vi "Parallel Event Init.vi"(5 "stop":refnum<vi>, 6 "parent":refnum<vi>, 7 "error in":errorcluster, 8 "max PVs per thread":i32=100, 9 "field names":string[](array[string]), 10 "PV names":string[](array[string])) -> (0 "error out":errorcluster, 1 "number of threads":i32, 2 "references of results":T1(array[cluster]), 3 "subVI References":cluster{refnum<vi>[], refnum<vi>[]})   [LabVIEW 2019]
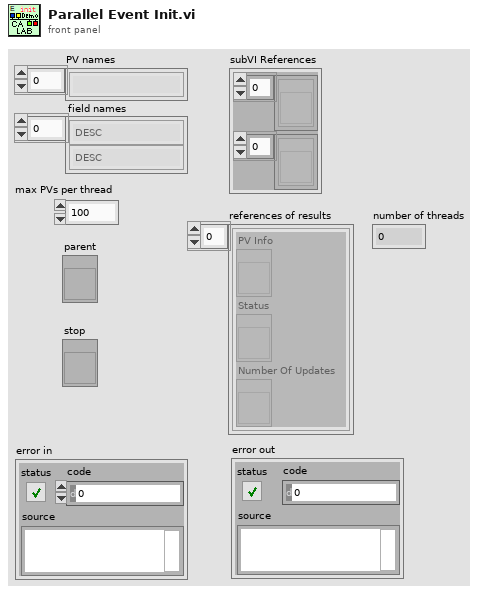
[diagram p1: front panel]
types:
  T1 = cluster{"PV Info":refnum<vi>, "Status":refnum<vi>, "Number Of Updates":refnum<vi>}[]
  T2 = map{string, cluster{"PV Info":refnum<vi>, "Status":refnum<vi>, "Number Of Updates":refnum<vi>}}
  T3 = cluster{"PV Info":refnum<vi>, "Status":refnum<vi>, "Number Of Updates":refnum<vi>}
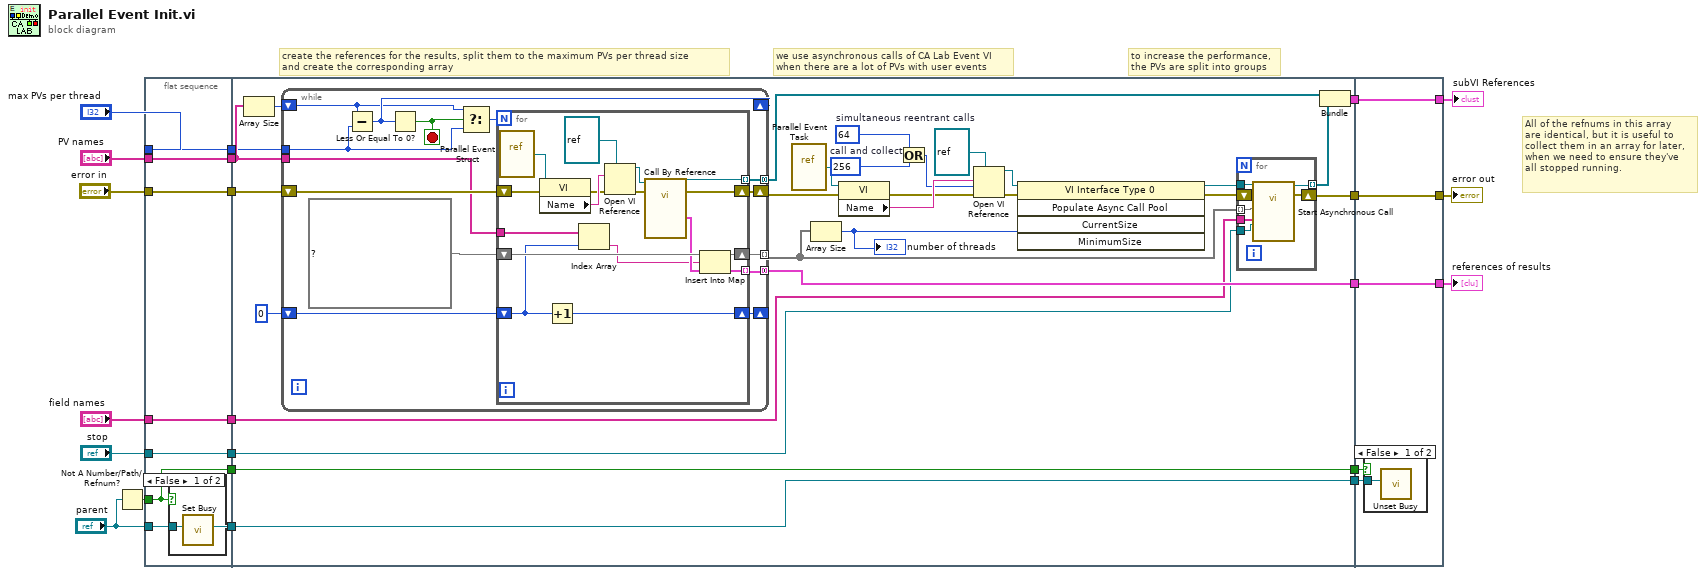
[diagram p0: block diagram]
diagram:
  # "All of the refnums in this array\nare identical, but it is useful to\ncollect them in an array for later,\nwhen we need to ensure they've\nall stopped running."
  # "create the references for the results, split them to the maximum PVs per thread size\nand create the corresponding array"
  # "to increase the performance,\nthe PVs are split into groups"
  # "we use asynchronous calls of CA Lab Event VI\nwhen there are a lot of PVs with user events"
  n1 = Not A Number/Path/Refnum?(number/path/refnum="parent") -> (NaN/Path/Refnum?=w3:bool)
  n2 = flat-sequence {
    tunnel: "field names" -> [w25]
    tunnel: "stop" -> [w26]
    tunnel: "max PVs per thread" -> [w27]
    tunnel: "PV names" -> [w28]
    tunnel: "error in" -> [w29]
    tunnel: [w29] -> w14
    tunnel: [w28] -> w13
    tunnel: [w27] -> w12
    tunnel: [w26] -> w11
    tunnel: [w25] -> w10
    tunnel: "parent" -> [w24]
    tunnel: [w24] -> w5
    tunnel: w3 -> [w23]
    tunnel: [w23] -> w1
    tunnel: w14 -> [w58]
    tunnel: w13 -> [w40]
    tunnel: w12 -> [w38]
    tunnel: w11 -> [w37]
    tunnel: w10 -> [w35]
    tunnel: [w43] -> w9
    tunnel: [w42] -> w8
    tunnel: [w33] -> w7
    tunnel: [w32] -> w6
    tunnel: w5 -> [w32]
    tunnel: [w31] -> w2
    tunnel: w1 -> [w31]
    tunnel: [w98] -> w15
    tunnel: [w99] -> w20
    tunnel: [w100] -> w21
    tunnel: w9 -> [w100]
    tunnel: w8 -> [w99]
    tunnel: w7 -> [w98]
    tunnel: w6 -> [w97]
    tunnel: w2 -> [w96]
    frame #0 {
      n3 = case shown="False" w23 {
        tunnel: w24 -> [w30 _]
        frame False {
          n4 = call <vilib>:"Set Busy.vi"("VI reference (current VI)"=w30) -> ()  [unwired: 9 in, 2 out]
        }
        frame True {
        }
      }
    }
    frame #1 {
      w48 = 256  # call and collect
      w49 = 64  # simultaneous reentrant calls
      n5 = Array Size(array=w40) -> (size(s)=w39:i32)
      n6 = while {
        tunnel: [w78] -> w36 mode=concatenating
        shift-right: [w77] -> w34
        shift-left: w58 -> [w79]
        tunnel: [w76] -> w44 mode=indexing
        shift-right: [w74] -> _
        shift-left: 0 -> [w75]
        shift-right: [w70] -> _
        shift-left: w39 -> [w68]
        tunnel: [w72] -> w43 mode=concatenating
        tunnel: w40 -> [w67]
        tunnel: w38 -> [w66]
        stop <- w69 stop-if-true
        n7 = Subtract(x=w68, y=w66) -> (x-y=w70:i32)
        n8 = Less Or Equal To 0?(x=w70) -> (x <= 0?=w69:bool)
        n9 = Select(t=w68, s=w69, f=w66) -> (s? t:f=w71:i32)
        n10 = for {
          N: w71 -> [_]
          tunnel: [w89] -> w78 mode=indexing
          shift-right: [w88] -> w77
          shift-left: w79 -> [w87]
          shift-right: [w86] -> w76
          shift-left: T2 {} ("map in") -> [w85]
          shift-right: [w80] -> w74
          shift-left: w75 -> [w83]
          tunnel: [w84] -> w72 mode=indexing
          tunnel: w67 -> [w81]
          n11 = vi-ref "Parallel Event Struct.vi"() -> (w95:refnum<vi>)
          n12 = property class="VI"(reference=w95, error in=w87) -> (error out=w90:errorcluster, "Name"=w94:string)  [unwired: 1 out]
          n13 = Increment(x=w83) -> (x+1=w80:i32)
          n14 = Index Array(array=w81, index=w83) -> (element=w82:string)
          n15 = Open VI Reference(type specifier VI Refnum (for type only)=refnum<vi> refnum, vi path=w94, error in (no error)=w90) -> (vi reference=w92:refnum<vi>, error out=w91:errorcluster)  [unwired: 3 in]
          n16 = call-by-ref "?"(reference=w92, error in=w91) -> (reference out=w89:refnum<vi>, error out=w88:errorcluster, "References"=w84:T3)
          n17 = Insert Into Map(map in=w85, key=w82, value=w84) -> (map out=w86:T2)  [unwired: 2 out]
        }
      }
      n18 = vi-ref "Parallel Event Task.vi"() -> (w56:refnum<vi>)
      n19 = Array Size(array=w44) -> (size(s)=w50:i32)
      "number of threads" <- w50
      n20 = property class="VI"(reference=w56, error in=w34) -> (error out=w54:errorcluster, "Name"=w55:string)  [unwired: 1 out]
      n21 = Or(x=w49, y=w48) -> (x .or. y?=w47:i32)
      n22 = Open VI Reference(type specifier VI Refnum (for type only)=refnum<vi> refnum, vi path=w55, options=w47, error in (no error)=w54) -> (vi reference=w51:refnum<vi>, error out=w52:errorcluster)  [unwired: 2 in]
      n23 = invoke class="VI Interface Type 0" method="Populate Async Call Pool"(reference=w51, error in=w52, "MinimumSize"=w50) -> (reference out=w46:refnum<vi>, error out=w45:errorcluster)  [unwired: 2 in, 3 out]
      n24 = for {
        tunnel: w44 -> [w63] mode=indexing
        tunnel: w35 -> [w62]
        tunnel: w37 -> [w61]
        shift-right: [w60] -> w42
        shift-left: w45 -> [w64]
        tunnel: w46 -> [w65]
        tunnel: [w59] -> w41 mode=indexing
        n25 = call-by-ref "Start Asynchronous Call"(reference=w65, error in=w64, "Stop reference"=w61, "Field Names"=w62, "map of references"=w63) -> (reference out=w59:refnum<vi>, error out=w60:errorcluster)  [unwired: 9 in]
      }
      n26 = Bundle(w36, w41) -> (w33:cluster{refnum<vi>[], refnum<vi>[]})  [unwired: 1 in]
    }
    frame #2 {
      n27 = case shown="False" w96 {
        tunnel: w97 -> [w101 _]
        frame False {
          n28 = call <vilib>:"Unset Busy.vi"("VI reference (current VI)"=w101) -> ()  [unwired: 10 in, 1 out]
        }
        frame True {
        }
      }
    }
  }
  "references of results" <- w21
  "error out" <- w20
  "subVI References" <- w15
